vi "Step 3 - Analyze Quantized Decimation (NStageMRate).vi"() -> ()   [LabVIEW 2023]
doc: "Demonstrates how to use the Multistage Multirate Filter Design Express VI to design a multistage decimation filter and then use this Express VI to quantize the coefficients of the multistage decimation filter. The examples also demonstrates how to use the DFD Plot NStage MRate Freq Response VI to analyze the characteristics of the quantized decimation filter."
uses:
  <vilib>/addons/Digital Filter Design/NI_DigFilterLicensed.lvlib
panel:
  in  "Stage View":u16(ring) items=["Overall", "Stage 1", "Stage 2", "Stage 3"]
  out "Magnitude Response":cluster{"f0":dbl, "df":dbl, "values":dbl[]}[](graph)
  # "Select Help>>Show Context Help and move the cursor over the VI icon for more information."
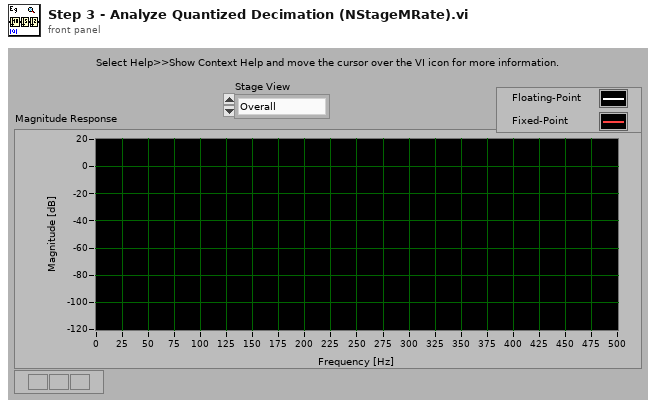
[diagram p1: front panel]
types:
  T1 = typedef "NI_DigFilterLicensed.lvlib/DFD Multirate Filter Obj.ctl" = cluster{"mMRate_Structure":enum16{"CIC", "FIR", "IIR", "Lattice"}, "mMRate_Mode":T2, "mMRate_Factor":i32, "mMRate_FIRParams":cluster{"mMRate_FIR_H":dbl[], "mMRate_FIR_IsNyquist?":bool, "mMRate_FIR_IsSymmetric?":bool}, "mMRate_CICParams":cluster{"mMRate_CIC_#Stage":i32, "mMRate_CIC_Lag":i32, "mMRate_CIC_Type":enum16{"Lowpass", "Highpass"}}, "mMRate_Order":i32, "mMRate_Version":string, "mMRate_Comments":string, "mMRate_RationalFactor":cluster{"mMRate_L":i32, "mMRate_M":i32}, "mMRate_Fs":dbl, "mMRate_Quantized?":bool, "mMRate_QFilterGain":dbl, "mMRate_CoefWl":i16, "mMRate_Scaling":cluster{"mMRate_ScaleByPowerOf2?":bool, "mMRate_ScaleType":T3}, "mMRate_InputWl":i16, "mMRate_OutputWl":i16, "mMRate_OutputMode":T4, "mMRate_MultMode":T5, "mMRate_BitPruning":bool, "mMRate_GainWl":i16, "mMRate_OutputFwl":i16, "mMRate_SumIwl":i16, "mMRate_InputIwl ":i16, "mMRate_SumWl":i16, "mMRate_CoefIwl":i16}
  T2 = typedef "NI_DigFilterLicensed.lvlib/DFD Multirate Mode.ctl" = i16
  T3 = typedef "NI_DigFilterLicensed.lvlib/DFD Coef Norm Type.ctl" = enum16{"No Norm", "Time Domain 1-Norm", "Time Domain 2-Norm", "Time Domain Inf-Norm"}
  T4 = typedef "NI_DigFilterLicensed.lvlib/DFD Round-off Mode.ctl" = enum16{"Nearest", "Truncation"}
  T5 = typedef "NI_DigFilterLicensed.lvlib/DFD FXP MRate Multiply Mode.ctl" = enum16{"Truncated", "Full"}
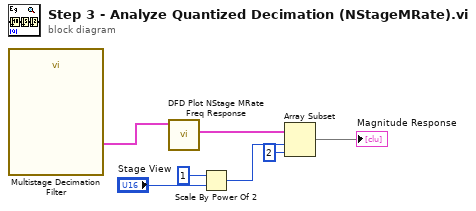
[diagram p0: block diagram]
diagram:
  n1 = call "Multistage Decimation Filter"() -> ("multirate filters out"=w1:T1[])  [unwired: 11 out]
  n2 = call <vilib>:"DFD Plot NStage MRate Freq Response.vi"("multirate filters in"=w1) -> ("magnitude responses"=w7:cluster{"f0":dbl, "df":dbl, "values":dbl[]}[])  [unwired: 6 in, 4 out]
  n3 = Scale By Power Of 2(n=1, x="Stage View") -> (x*2^n=w4:u16)
  n4 = Array Subset(array=w7, index=w4, length=2) -> (→"Magnitude Response":cluster{"f0":dbl, "df":dbl, "values":dbl[]}[])
